vi "PPMS.getTemperature.vi"(8 "error in (no error)":errorcluster, 11 "instrument.PPMS":refnum<class "instrument.PPMS.lvclass">) -> (0 "error out":errorcluster, 2 "Temperature Status":T1, 3 "instrument.PPMS out":refnum<class "instrument.PPMS.lvclass">)   [LabVIEW 2019, in "instrument.PPMS.lvclass"]
uses:
  instrument.PPMS.lvclass
  Typedefs/PPMS.Temperature Status--cluster.ctl
  instrument.PPMS.lvclass/instrument.PPMS.ctl
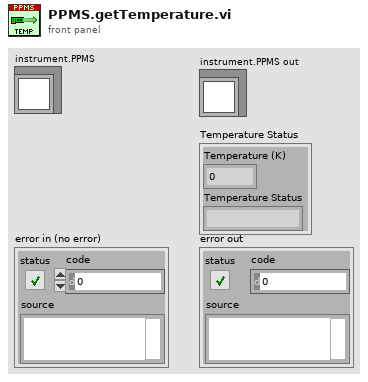
[diagram p1: front panel]
types:
  T1 = typedef "instrument.PPMS.lvclass/PPMS.Temperature Status--cluster.ctl" = cluster{"Temperature (K)":dbl, "Temperature Status":string}
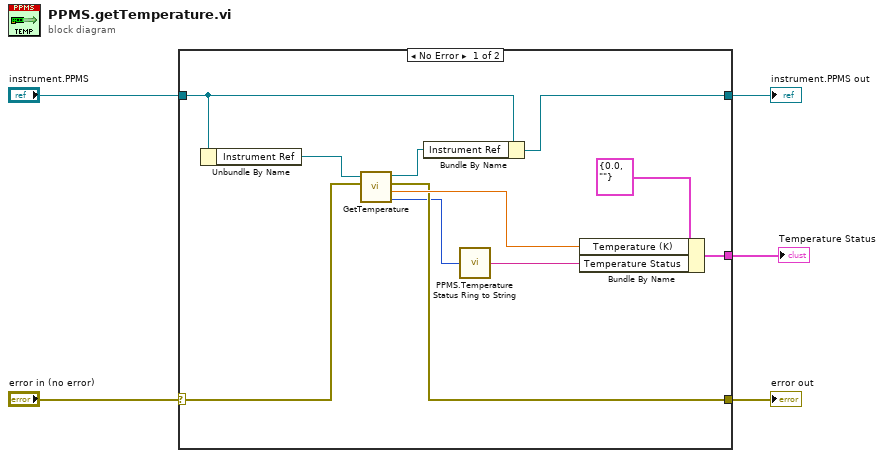
[diagram p0: block diagram]
diagram:
  n1 = case shown="No Error" "error in (no error)" {
    selector: "error in (no error)" -> [w14 w18]
    tunnel: [w12 w18] -> w5
    tunnel: "instrument.PPMS" -> [w8 w17]
    tunnel: [w9 w17] -> w2
    tunnel: [w16 _] -> w1
    frame No Error {
      n2 = Unbundle By Name(w8) -> ("Instrument Ref"=w11:refnum<k24>)
      n3 = call "GetTemperature.vi"("error in (no error)"=w14, "Instrument Ref In"=w11) -> ("Temperature\nStatus"=w7:i32, "Temperature"=w13:dbl, "error out"=w12:errorcluster, "Instrument Ref Out"=w10:refnum<k24>)  [unwired: 3 in, 1 out]
      n4 = Bundle By Name(cluster=w8, "Instrument Ref"=w10) -> (w9:refnum<class "instrument.PPMS.lvclass">)
      n5 = call "PPMS.Temperature Status Ring to String.vi"("Temperature Status"=w7) -> ("Status String"=w6:string)
      n6 = Bundle By Name(cluster=T1 {"Temperature (K)"=0.0, "Temperature Status"=""} ("Temperature Status"), "Temperature (K)"=w13, "Temperature Status"=w6) -> (w16:T1)
    }
    frame Error {
    }
  }
  "Temperature Status" <- w1
  "error out" <- w5
  "instrument.PPMS out" <- w2
